vi "compute_engine_CH0CH1_Rev01.vi"(0 "INPUT 1L Loc":dbl step=0.001, 1 "INPUT 2R Loc":dbl step=0.001, 3 "Array In":u8[](array[numeric]), 4 "Input Select":u16(ring), 5 "Control Character":string, 8 "Divider INPUT1L":dbl, 9 "Number of datapoints":dbl, 12 "Divider INPUT2R":dbl, 13 "DC Filter":bool, 14 "Shift INPUT 1L":dbl, 15 "AC/DC INPUT2":bool, 16 "Shift INPUT 2R":dbl, 19 "AC /DC INPUT1":bool) -> (10 "INPUT2":dbl[](array[numeric]), 17 "VRMS INPUT1":dbl format="%#.6g", 18 "INPUT1":dbl[](array[numeric]), 20 "VDC INPUT2":dbl format="%#.6g", 21 "VRMS INPUT2":dbl format="%#.6g", 23 "Freq CH1 Hz":dbl format="%#.6g", 24 "VDC INPUT1":dbl format="%#.6g", 25 "Freq CH0 Hz":dbl format="%#.6g", 26 "Sig Out":dynamicdata(graph), 27 "RAW":dynamicdata(graph))   [LabVIEW 2012]
panel:
  out "CH1_OUT":dbl[](graph)
  out "CH0_OUT":dbl[](graph)
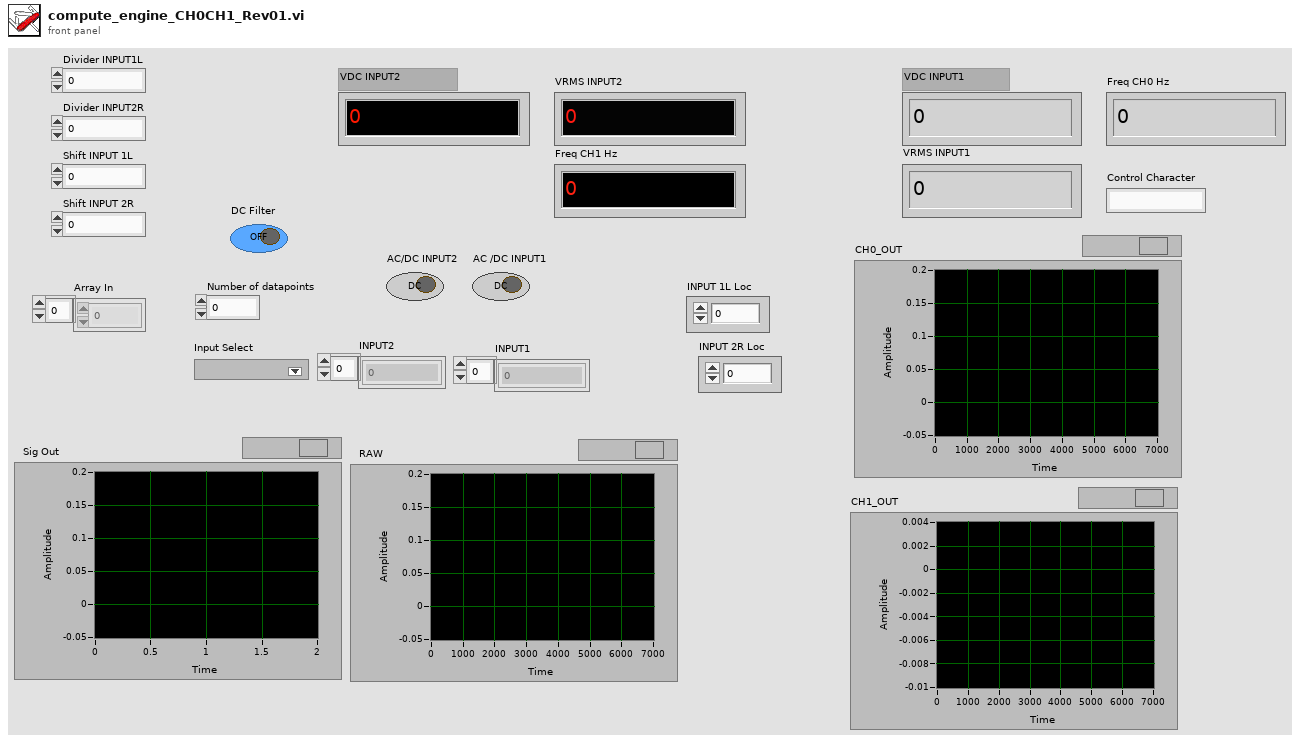
[diagram p1: front panel]
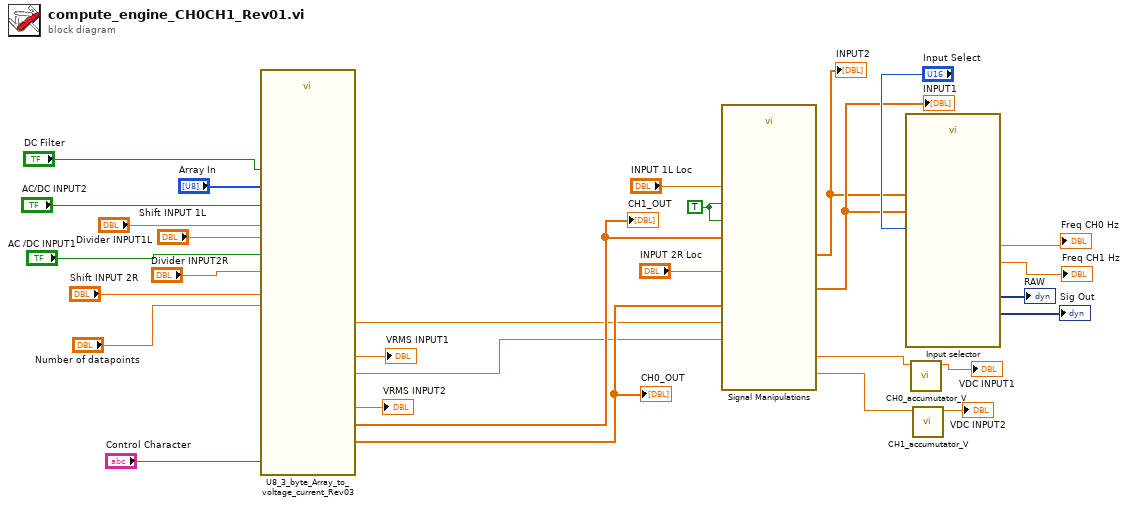
[diagram p0: block diagram]
diagram:
  w29 = TRUE
  n1 = call "U8_3_byte_Array_to_voltage_current_Rev03.vi"("Nmbr_of_datapoints"="Number of datapoints", "Array In"="Array In", "INPUT1 AC couple"="AC/DC INPUT2", "INPUT2 AC couple"="AC /DC INPUT1", "Div INPUT 2R"="Divider INPUT2R", "Div INPUT 1L"="Divider INPUT1L", "Shift INPUT 2R"="Shift INPUT 2R", "Control Character"="Control Character", "AC/DC"="DC Filter", "Shift INPUT 1L"="Shift INPUT 1L") -> ("INPUT1RMS"=→"VRMS INPUT1":dbl, "INPUT2RMS"=→"VRMS INPUT2":dbl, "INPUT1 Vave"=w6:dbl, "INPUT2 Vave"=w3:dbl, "INPUT 1L"=w27:dbl[], "INPUT 2R"=w26:dbl[])  [unwired: 2 in, 2 out]
  "CH0_OUT" <- w27
  "CH1_OUT" <- w26
  n2 = call "Signal Manipulations.vi"("INPUT1 Differential Mode"=w29, "VDC INPUT2"=w3, "INPUT2 Differential Mode"=w29, "VDC INPUT1"=w6, "INPUT 2R Loc"="INPUT 2R Loc", "INPUT 2R Line In"=w26, "INPUT 1L Loc"="INPUT 1L Loc", "INPUT 1L Line In"=w27) -> ("VDC INPUT2"=w2:dbl, "VDC INPUT1"=w5:dbl, "INPUT1L Line Out"=w12:dbl[], "INPUT2R Line Out"=w11:dbl[])
  "INPUT2" <- w11
  "INPUT1" <- w12
  n3 = call "Input selector.vi"("Voltage INPUT2"=w12, "Voltage INPUT1"=w11, "Ring"="Input Select") -> ("INPUT2 (Hz)"=→"Freq CH1 Hz":dbl, "INPUT1 (Hz)"=→"Freq CH0 Hz":dbl, "Sig Out"=→"Sig Out":dynamicdata, "RAW"=→"RAW":dynamicdata)  [unwired: 3 in, 2 out]
  n4 = call "CH0_accumutator_V.vi"("Vin"=w5) -> ("voltage_acc"=→"VDC INPUT1":dbl)  [unwired: 10 in]
  n5 = call "CH1_accumutator_V.vi"("Vin"=w2) -> ("voltage_acc"=→"VDC INPUT2":dbl)  [unwired: 10 in]
